vi "Vision_Test2.vi"() -> ()   [LabVIEW 2011]
panel:
  in  "Threshold Range":cluster{"Lower value":sgl, "Upper value":sgl}={"Lower value"=240.0, "Upper value"=255.0}
  in  "Milsec Wait":u32=5000
  in  "Take Pics":bool
  out "Image 2":T1(plugin-control)
  out "Image 1":T1(plugin-control)
  out "Binary Image 2":T1(plugin-control)
  out "Binary Image 1":T1(plugin-control)
  out "Processed Image":T1(plugin-control)
  out "Offset Angle From Perpendicular":dbl
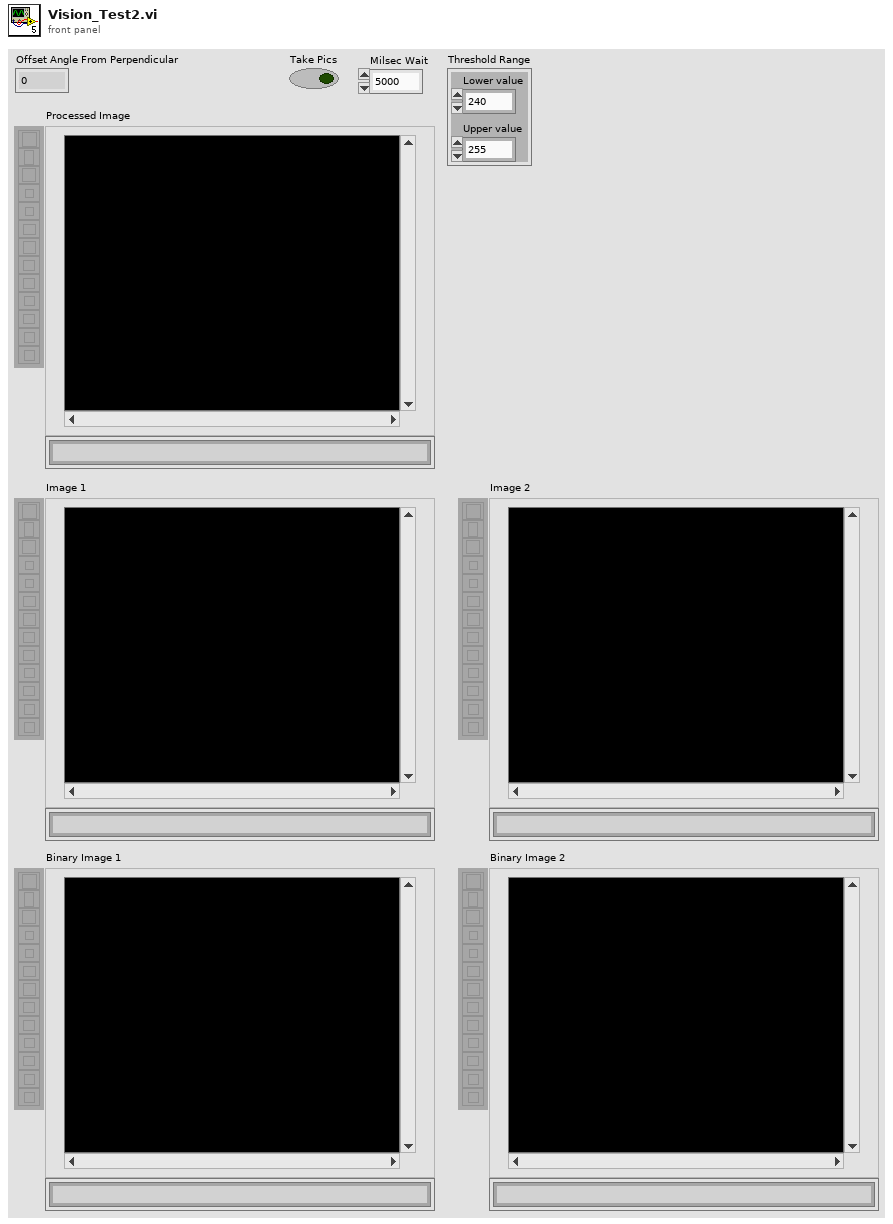
[diagram p1: front panel]
types:
  T1 = typedef "IMAQ Image.ctl" = refnum<image>
  T2 = typedef "WPI_CameraDevRef.ctl" = cluster{"Camera Address":string, "CameraStatus":errorcluster, "Acquire Image Notifier":refnum<notifier>}
  T3 = cluster{"Image_Dsts_Out[0]":T1, "Image_Dsts_Out[1]":T1, "Image_Dsts_Out[2]":T1, "Image_Dsts_Out[3]":T1, "Image_Dsts_Out[4]":T1, "Image_Dsts_Out[5]":T1, "Image_Dsts_Out[6]":T1, "Image_Dsts_Out[7]":T1, "Image_Dsts_Out[8]":T1}
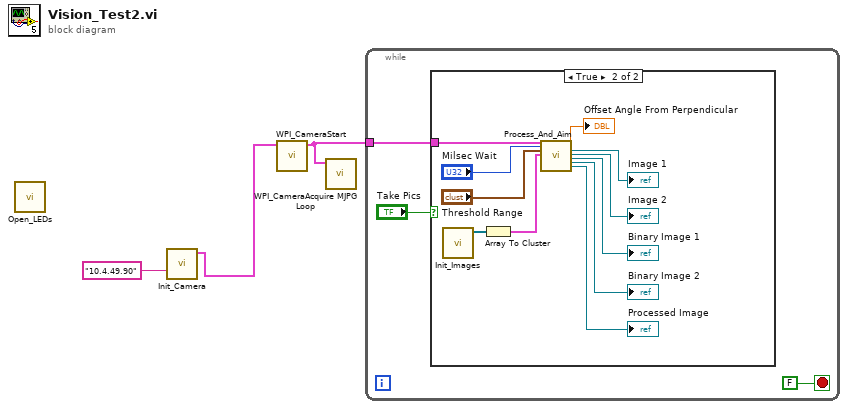
[diagram p0: block diagram]
diagram:
  n1 = call "Open_LEDs.vi"() -> ()  [unwired: 11 in, 1 out]
  n2 = call "Init_Camera.vi"("Camera IP"="10.4.49.90") -> ("CameraDevRef Out"=w1:T2)  [unwired: 10 in]
  n3 = call <vilib>:"WPI_CameraStart.vi"("CameraDevRef"=w1) -> ("CameraDevRef Out"=w3:T2)  [unwired: 9 in, 1 out]
  n4 = call <vilib>:"WPI_CameraAcquire MJPG Loop.vi"("CameraDevRef"=w3) -> ()  [unwired: 11 in]
  n5 = while {
    tunnel: w3 -> [w6]
    stop <- FALSE stop-if-true
    n6 = case shown="True" "Take Pics" {
      tunnel: w6 -> [_ w17]
      frame False {
      }
      frame True {
        n7 = call "Init_Images.vi"() -> ("Image_Dsts_Out"=w8:T1[])  [unwired: 11 in]
        n8 = Array To Cluster(array=w8) -> (cluster=w7:T3)
        n9 = call "Process_And_Aim.vi"("CameraDevRef"=w17, "Milsec Wait"="Milsec Wait", "Threshold Range"="Threshold Range", "Image Dsts Clust"=w7) -> ("Offset Angle From Perpendicular"=→"Offset Angle From Perpendicular":dbl, "Image 1 Out"=→"Image 1":T1, "Image 2 Out"=→"Image 2":T1, "Binary 1 Out"=→"Binary Image 1":T1, "Binary 2 Out"=→"Binary Image 2":T1, "Processed Image Out"=→"Processed Image":T1)  [unwired: 17 in, 1 out]
      }
    }
  }
